vi "Parse Structure IDs.vi"(8 "Error In":errorcluster, 9 "Data":string, 11 "Nest Config":T1) -> (0 "Error Out":errorcluster, 1 "Data":string, 2 "Structure IDs":string[](array[string]), 3 "Nest Config":T1)   [LabVIEW 2013, in "LVH-Nest.lvlib"]
doc: "Get structure IDs."
uses:
  LVH-Nest.lvlib
  Type Defs/Nest Config.ctl
  <vilib>/httpClient/ClientHandle.ctl
  Type Defs/Session Data.ctl
  <vilib>/httpClient/LabVIEWHTTPClient.lvlib
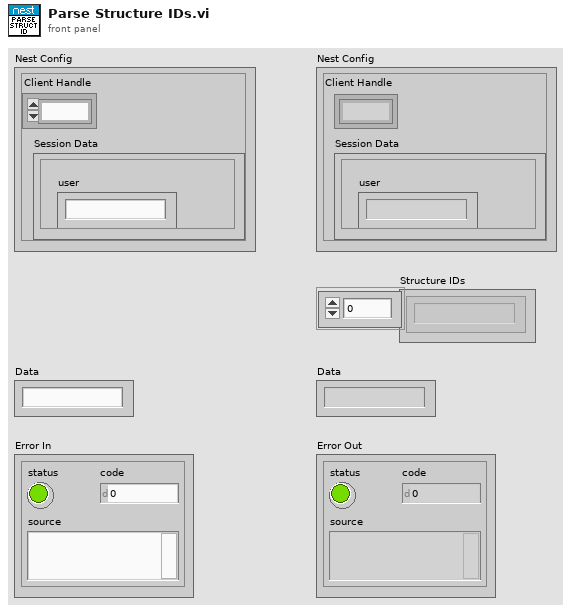
[diagram p1: front panel]
types:
  T1 = typedef "LVH-Nest.lvlib/Nest Config.ctl" = cluster{"Client Handle":T2, "Session Data":T3}
  T2 = typedef "LabVIEWHTTPClient.lvlib/ClientHandle.ctl" = refnum<k1>
  T3 = typedef "LVH-Nest.lvlib/Session Data.ctl" = cluster{"is_superuser":bool, "is_staff":bool, "urls":cluster{"transport_url":string, "rubyapi_url":string, "weather_url":string, "log_upload_url":string, "support_url":string}, "limits":cluster{"thermostats_per_structure":u32, "structures":u32, "thermostats":u32, "smoke_detectors":u32, "smoke_detectors_per_structure":u32}, "access_token":string, "userid":string, "expires_in":string, "email":string, "user":string, "language":string}
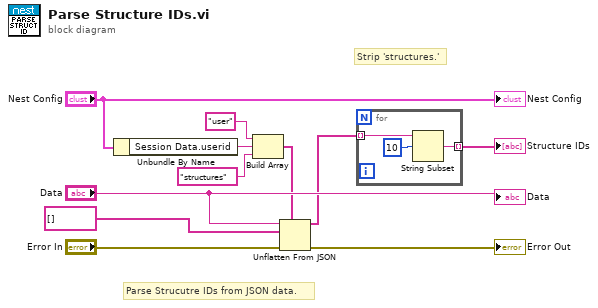
[diagram p0: block diagram]
diagram:
  # "Strip 'structures.'"
  # "Parse Strucutre IDs from JSON data."
  n1 = Unbundle By Name("Nest Config") -> ("Session Data.userid"=w5:string)
  n2 = Build Array("user", w5, "structures" ("element")) -> (w7:string[])
  n3 = Unflatten From JSON(path=w7, JSON string="Data", type and defaults=string[] [], error in (no error)="Error In") -> (value=w2:string[], error out=→"Error Out":errorcluster)  [unwired: 3 in]
  n4 = for {
    tunnel: w2 -> [w13] mode=indexing
    tunnel: [w12] -> w1 mode=indexing
    n5 = String Subset(string=w13, offset (0)=10) -> (substring=w12:string)  [unwired: 1 in]
  }
  "Structure IDs" <- w1
  "Data" <- "Data"
  "Nest Config" <- "Nest Config"
